vi "Generate DO Finite Pulses.vi"(8 "error in":errorcluster, 10 "DO Finite Pulse Config":T1={"Port Number"=0, "Number of Pulses"=20, "High Time (ms)"=20, "Low Time (ms)"=20}, 11 "DUT Sample in":refnum<class "DUT Sample.lvclass">) -> (0 "error out":errorcluster, 3 "DUT Sample out":refnum<class "DUT Sample.lvclass">)   [LabVIEW 2023, in "DUT Sample.lvclass"]
uses:
  DUT Sample.lvclass
  DUT Sample.lvclass/DUT Sample.ctl
  <resource>/objmgr/daqmx.rc
  <vilib>/DAQmx/configure/timing.llb/DAQmx Timing (Implicit).vi
  <vilib>/DAQmx/create/channels.llb/DAQmx Create Channel (CO-Pulse Generation-Time).vi
  typedefs/DO Finite Pulse Config.ctl
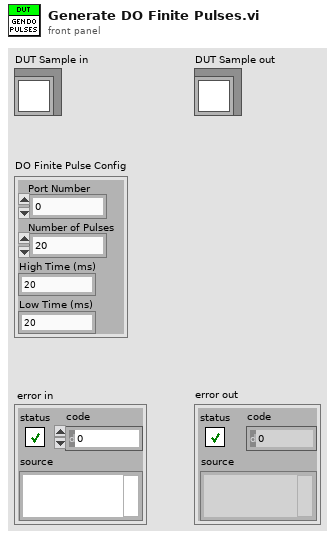
[diagram p1: front panel]
types:
  T1 = typedef "DUT Sample.lvclass/DO Finite Pulse Config.ctl" = cluster{"Port Number":u8, "Number of Pulses":u8, "High Time (ms)":u16, "Low Time (ms)":u16}
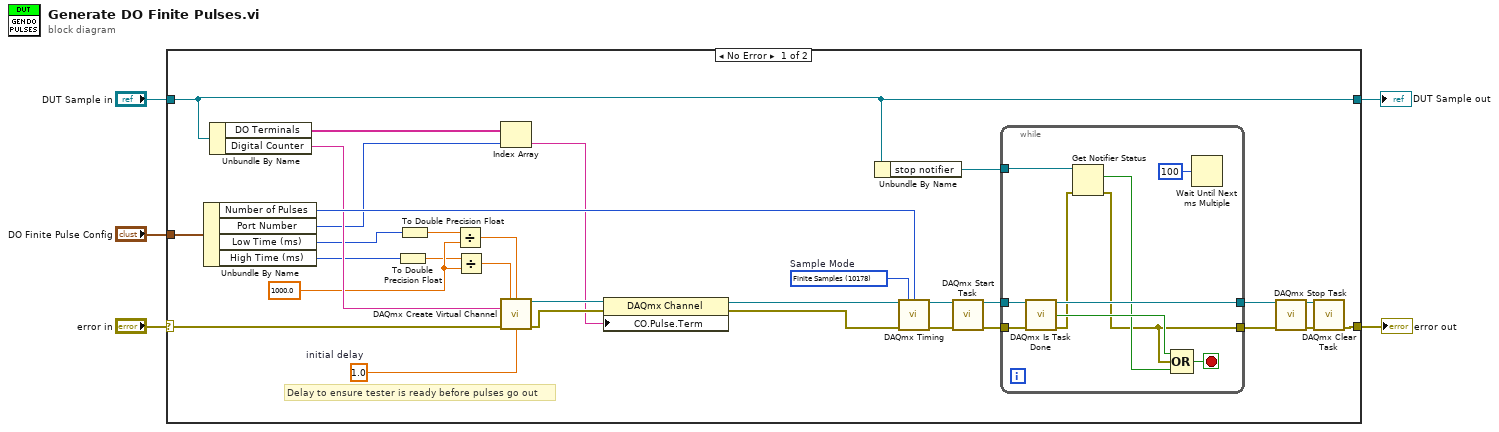
[diagram p0: block diagram]
diagram:
  n1 = case shown="No Error" "error in" {
    selector: "error in" -> [w20 w48]
    tunnel: "DO Finite Pulse Config" -> [w23 _]
    tunnel: [w21 w48] -> w4
    tunnel: "DUT Sample in" -> [w18 w47]
    tunnel: [w18 w47] -> w1
    frame No Error {
      w6 = 1.0  # initial delay
      w11 = 1000.0 ("y")
      w36 = 10178 items=["Finite Samples"=10178, "Continuous Samples"=10123, "Hardware Timed Single Point"=12522]  # Sample Mode
      # "Delay to ensure tester is ready before pulses go out"
      n2 = Unbundle By Name(w23) -> ("Number of Pulses"=w22:u8, "Port Number"=w15:u8, "Low Time (ms)"=w10:u16, "High Time (ms)"=w13:u16)
      n3 = Unbundle By Name(w18) -> ("DO Terminals"=w16:tag[], "Digital Counter"=w17:tag)
      n4 = To Double Precision Float(number=w13) -> (double precision float=w7:dbl)
      n5 = To Double Precision Float(number=w10) -> (double precision float=w8:dbl)
      n6 = Divide(x=w8, y=w11) -> (x/y=w9:dbl)
      n7 = Divide(x=w7, y=w11) -> (x/y=w12:dbl)
      n8 = Index Array(array=w16, index=w15) -> (element=w14:tag)
      n9 = call-poly <vilib>:"DAQmx Create Virtual Channel.vi"("high time"=w12, "low time"=w9, "counter"=w17, "error in"=w20, "initial delay"=w6) -> ("task out"=w31:refnum<k21>, "error out"=w30:errorcluster)  [unwired: 9 in]
      n10 = property on="Property Node" class="DAQmx Channel"(reference=w31, error in=w30, "CO.Pulse.Term"=w14) -> (reference out=w28:refnum<k21>, error out=w29:errorcluster)
      n11 = Unbundle By Name(w18) -> ("stop notifier"=w19:refnum<notifier>)
      n12 = call-poly <vilib>:"DAQmx Timing.vi"("task/channels in"=w28, "sample mode"=w36, "samples per channel"=w22, "error in"=w29) -> ("task out"=w32:refnum<k21>, "error out"=w33:errorcluster)  [unwired: 10 in]
      n13 = call <vilib>:"DAQmx Start Task.vi"("task/channels in"=w32, "error in"=w33) -> ("task out"=w35:refnum<k21>, "error out"=w34:errorcluster)  [unwired: 12 in]
      n14 = while {
        tunnel: w35 -> [w46]
        tunnel: w34 -> [w45]
        tunnel: [w37] -> w24
        tunnel: [w43] -> w25
        tunnel: w19 -> [w40]
        stop <- w44 stop-if-true
        n15 = call <vilib>:"DAQmx Is Task Done.vi"("task/channels in"=w46, "error in"=w45) -> ("task out"=w43:refnum<k21>, "task done?"=w41:bool, "error out"=w38:errorcluster)  [unwired: 11 in]
        n16 = Get Notifier Status(notifier=w40, error in (no error)=w38) -> (current notification=w39:bool, error out=w37:errorcluster)  [unwired: 3 out]
        n17 = Compound Arithmetic op=OR(w41, w37, w39) -> (w44:bool)
        n18 = Wait Until Next ms Multiple(millisecond multiple=u32 100) -> ()  [unwired: 1 out]
      }
      n19 = call <vilib>:"DAQmx Stop Task.vi"("task/channels in"=w25, "error in"=w24) -> ("task out"=w27:refnum<k21>, "error out"=w26:errorcluster)  [unwired: 12 in]
      n20 = call <vilib>:"DAQmx Clear Task.vi"("task in"=w27, "error in"=w26) -> ("error out"=w21:errorcluster)  [unwired: 13 in]
    }
    frame Error {
    }
  }
  "error out" <- w4
  "DUT Sample out" <- w1
